vi "To Variant.vi"(8 "Error In":errorcluster, 11 "TD String":refnum<class "String.lvclass">) -> (0 "Error Out":errorcluster, 2 "Variant":variant)   [LabVIEW 2020, in "NI_VIAnCFGDataStructure.lvlib" / "String.lvclass"]
doc: "Dynamic dispatch interface for conversion of Tree Data classes to variant LV data."
uses:
  <vilib>/addons/analyzer/VIAnCFGDataStructure/Data Types/String/String.lvclass
  <vilib>/addons/analyzer/VIAnCFGDataStructure/Data Types/String/String.lvclass/String.ctl
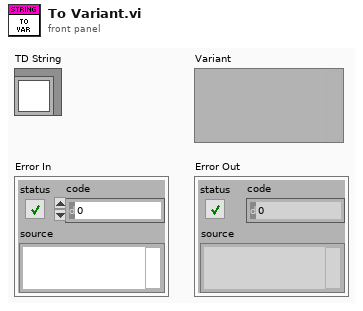
[diagram p1: front panel]
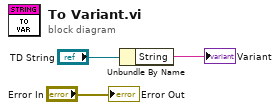
[diagram p0: block diagram]
diagram:
  n1 = Unbundle By Name("TD String") -> ("String"=→"Variant":string)
  "Error Out" <- "Error In"
